vi "Plug_In_Move_Trav_and_Meas.vi"() -> (5 "Plug in titles":string[](array[string]), 7 "Plug in values":string[](array[string]))   [LabVIEW 2010]
uses:
  Controls/Post_Process.ctl
  Controls/User_Specific_mode.ctl
  Gen Trav/Trav_mode.ctl
  Globals/Meas_global.vi
  Globals/Trav_pos_global.vi
  Globals/Dynamic_call_global.ph.vi
panel:
  out "Case Currently On":string
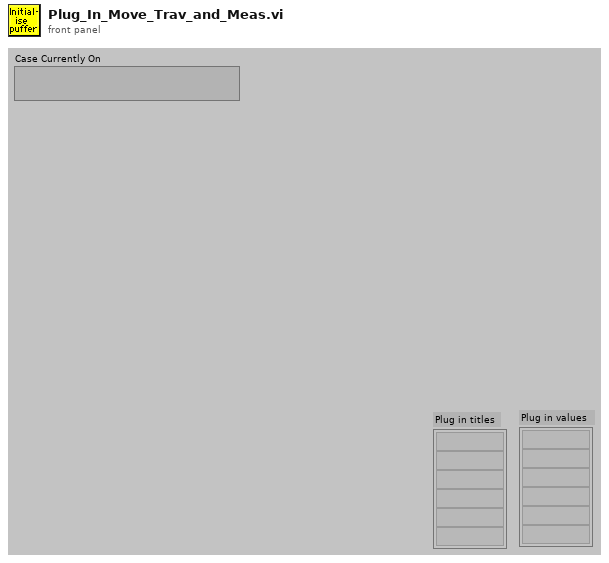
[diagram p1: front panel]
types:
  T1 = typedef "Traverse_cluster.ctl" = cluster{"Start X":dbl, "Start Y":dbl, "Start Z":dbl, "End X":dbl, "End Y":dbl, "End Z":dbl, "No. of pts.":i32, "Spacing":T2, "Filename":path, "Tunnel Speed":dbl, "Averaging time (min)":dbl, "Extra Commands":string, "Specific Arguments":string, "Emission Rate (l/min)":dbl, "Trace Gas Concentration (%)":dbl, "Density Ratio":string, "Comments":string, "Row No":i32, "Row Type Selector":T3, "Completion time":string, "Row Duration (mins)":dbl, "No. of Valid pts.":i32, "Meas Setup File":string}
  T2 = typedef "Spacing.ctl" = enum16{"Linear", "Log", "Gauss", "Specified", "N/A"}
  T3 = typedef "Multi_run_mode.ctl" = enum16{"Move Traverse Only", "Set Tunnel Speed Only", "Set Source Only", "Set Measurement Conditions", "Single Measurement", "Vertical Profile", "Lateral Profile", "Longitudinal Profile", "Explore Volume", "Multi-Axis Profile", "Auto Calibrate", "Meas Fast FID Bkgnd", "Check Beam Power", "Scanning Valve Measurement", "Run VI Named:", "Set ADAM Ch", "Wait (minutes)", "Send Message", "Synchronize With:", "Fall Back to this Row", "Turn Off Row Repeating", "Blank Row"}
  T4 = typedef "Post_Process.ctl" = enum16{"Take New Data", "Post Process Raw Data File"}
  T5 = typedef "User_Specific_mode.ctl" = enum16{"Check VI only", "Run VI"}
  T6 = typedef "Trav_mode.ctl" = enum16{"Move traverse", "Read traverse position", "Teach Position"}
  T7 = typedef "Rendezvous RefNum" = refnum<k1>
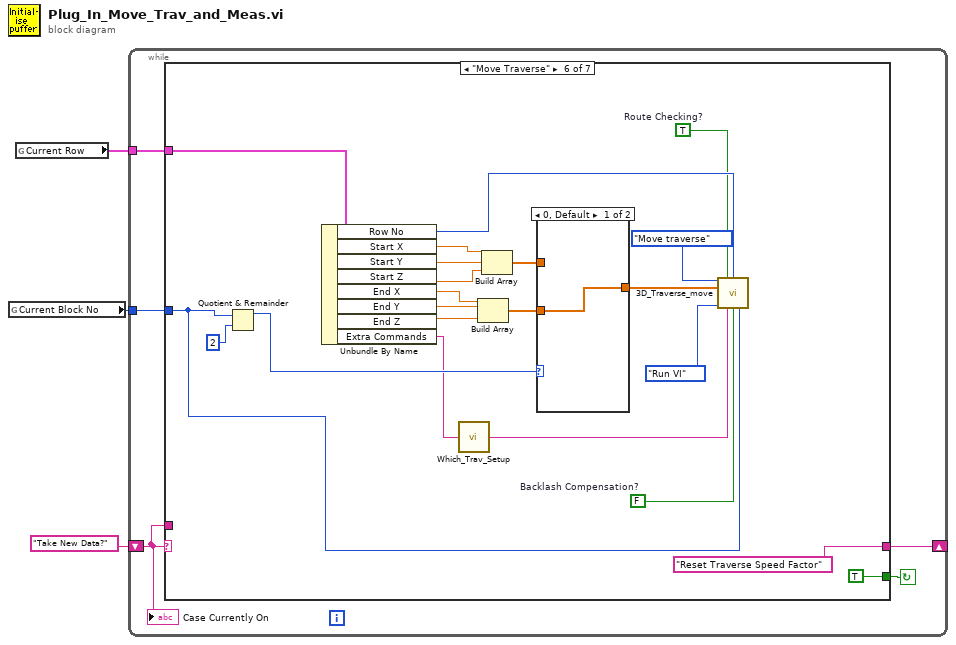
[diagram p0: block diagram]
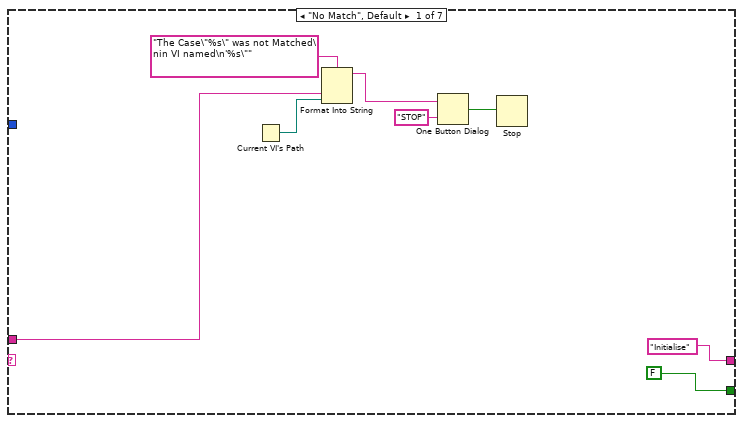
[diagram p2: hidden frame]
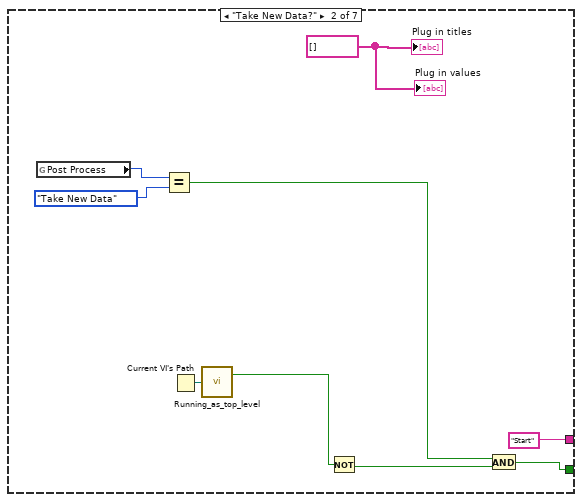
[diagram p3: hidden frame]
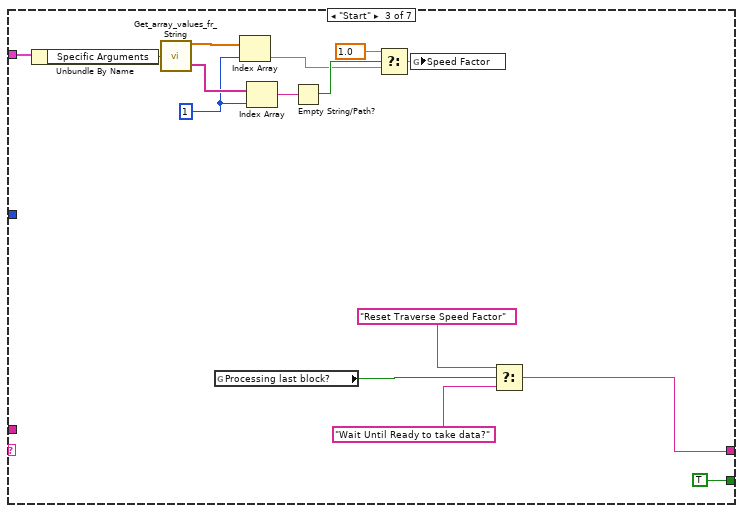
[diagram p4: hidden frame]
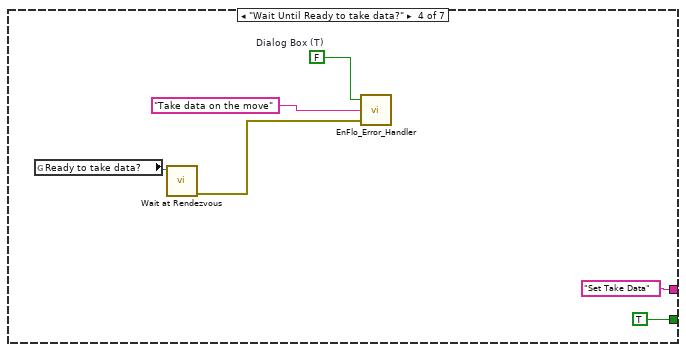
[diagram p5: hidden frame]
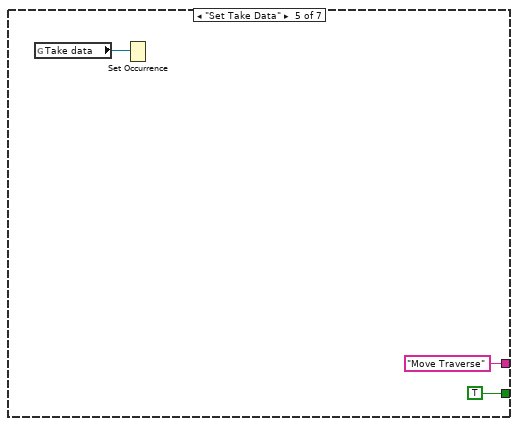
[diagram p6: hidden frame]
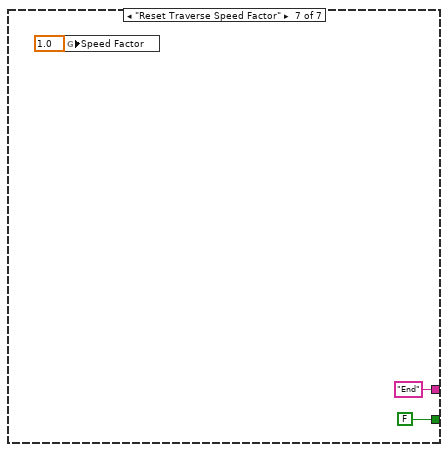
[diagram p8: hidden frame]
diagram:
  n1 = global read "Meas_global.vi" "Current Block No"() -> (w2:i32)
  n2 = global read "Trav_pos_global.vi" "Current Row"() -> (w1:T1)
  n3 = while {
    shift-left: "Take New Data?" -> [w6]
    shift-right: [w7] -> _
    tunnel: w2 -> [w5]
    tunnel: w1 -> [w4]
    stop <- w8 continue-if-true
    n4 = case shown="\"Move Traverse\"" w6 {
      tunnel: [FALSE w19 TRUE ("Command Found") TRUE ("Command Found") TRUE ("Command Found") TRUE ("Command Found") FALSE ("Command Found")] -> w8
      tunnel: ["Initialise" "Start" w29 "Set Take Data" "Move Traverse" "Reset Traverse Speed Factor" "End" ("f")] -> w7
      tunnel: w6 -> [w11 _ _ _ _ _ _]
      tunnel: w5 -> [_ _ _ _ _ w55 _]
      tunnel: w4 -> [_ _ w38 _ _ w53 _]
      frame "No Match", Default {
        n5 = Current VI's Path() -> (path=w10:path)
        n6 = Format Into String(format string="The Case\"%s\" was not Matched\nin VI named\n'%s\"" ("Format String"), w11, w10) -> (resulting string=w14:string)  [unwired: 2 in, 1 out]
        n7 = One Button Dialog(message=w14, button name ("OK")="STOP") -> (true=w12:bool)
        n8 = Stop(stop? (T)=w12) -> ()
      }
      frame "Take New Data?" {
        w22 = string[] [] ("Plug in titles")
        n9 = global read "Meas_global.vi" "Post Process"() -> (w24:T4)
        n10 = Equal?(x=w24, y=Post_Process."Take New Data" ("Post Process")) -> (x = y?=w20:bool)
        n11 = Current VI's Path() -> (path=w21:path)
        n12 = call "Running_as_top_level.vi"("Vi path name"=w21) -> ("Top Level"=w18:bool)  [unwired: 1 out]
        n13 = Not(x=w18) -> (.not. x?=w17:bool)
        n14 = And(x=w20, y=w17) -> (x .and. y?=w19:bool)
        "Plug in titles" <- w22
        "Plug in values" <- w22
      }
      frame "Start" {
        w27 = 1 ("index")
        n15 = Unbundle By Name(w38) -> ("Specific Arguments"=w40:string)
        n16 = call "Get_array_values_fr_String.vi"("String Value"=w40) -> ("Numeric Array"=w39:dbl[], "String array"=w37:string[])
        n17 = global read "Meas_global.vi" "Processing last block?"() -> (w31:bool)
        n18 = Index Array(array=w39, index=w27) -> (element=w34:dbl)
        n19 = Index Array(array=w37, index=w27) -> (element=w36:string)
        n20 = Empty String/Path?(string/path=w36) -> (empty?=w35:bool)
        n21 = Select(t=1.0, s=w35, f=w34) -> (s? t:f=w32:dbl)
        n22 = global write "Trav_pos_global.vi" "Speed Factor"(w32) -> ()
        n23 = Select(t="Reset Traverse Speed Factor" ("f"), s=w31, f="Wait Until Ready to take data?") -> (s? t:f=w29:string)
      }
      frame "Wait Until Ready to take data?" {
        w42 = FALSE  # Dialog Box (T)
        n24 = global read "Dynamic_call_global.ph.vi" "Ready to take data?"() -> (w45:T7)
        n25 = call <vilib>:"Wait at Rendezvous.vi"("rendezvous"=w45) -> ("error out"=w43:errorcluster)  [unwired: 4 in, 2 out]
        n26 = call "EnFlo_Error_Handler.vi"("error in (no error)"=w43, "Error Type"="Take data on the move", "Dialog Box (T)"=w42) -> ()  [unwired: 3 out]
      }
      frame "Set Take Data" {
        n27 = global read "Dynamic_call_global.ph.vi" "Take data"() -> (w47:refnum<k4>)
        n28 = Set Occurrence(w47) -> ()
      }
      frame "Move Traverse" {
        w50 = TRUE  # Route Checking?
        w68 = FALSE  # Backlash Compensation?
        n29 = Quotient & Remainder(x=w55, y=2) -> (x-y*floor(x/y)=w67:i32)  [unwired: 1 out]
        n30 = Unbundle By Name(w53) -> ("Row No"=w54:i32, "Start X"=w64:dbl, "Start Y"=w65:dbl, "Start Z"=w66:dbl, "End X"=w60:dbl, "End Y"=w59:dbl, "End Z"=w58:dbl, "Extra Commands"=w52:string)
        n31 = call "Which_Trav_Setup.vi"("Extra Command String"=w52) -> ("Traverse Setup"=w51:string)
        n32 = Build Array(w60, w59, w58) -> (w62:dbl[])
        n33 = Build Array(w64, w65, w66) -> (w61:dbl[])
        n34 = case shown="0, Default" w67 {
          tunnel: [w72 w73] -> w63
          tunnel: w62 -> [w72 _]
          tunnel: w61 -> [_ w73]
          frame 0, Default {
          }
          frame 1 {
          }
        }
        n35 = call "3D_Traverse_move.vi"("Mode"=Trav_mode."Move traverse", "Route Checking?"=w50, "Row Number"=w54, "Position"=w63, "Simulate/Run"=User_Specific_mode."Run VI", "Traverse name"=w51, "Backlash Compensation?"=w68, "Currently on Point"=w55) -> ()  [unwired: 5 in, 3 out]
      }
      frame "Reset Traverse Speed Factor" {
        n36 = global write "Trav_pos_global.vi" "Speed Factor"(1.0 ("Speed Factor")) -> ()
      }
    }
    "Case Currently On" <- w6
  }
